vi "Inflation Apparatus.vi"() -> ()   [LabVIEW 2020]
uses:
  Inflation Test/Controls/Open Loop Controls.ctl
  Inflation Test/Controls/Ramp Controls.ctl
  Inflation Test/Controls/sinusoidal controls.ctl
  Inflation Test/Controls/Blood Pressure Controls.ctl
  Inflation Test/Controls/Hardware Options.ctl
  <vilib>/userdefined/High Color/IMAQdx.ctl
  Inflation Test/Controls/Common IA Test Control.ctl
  Controller Loop/Message and Data.ctl
  Inflation Test/Parameter Class/IA Test Parameters.lvclass
  Controllers/Controller.lvclass
  Hardware/Sensors/Cameras/Camera.lvclass
  Hardware/Sensors/Force Sensors/Force Sensor.lvclass
  Hardware/Actuators/Servos/Servo.lvclass
  Hardware/Actuators/Switches/Switch.lvclass
  Hardware/Sensors/Cameras/Camera.lvclass/Camera.ctl
  GUI/Main GUI Loop/Handler.ctl
  Hardware/Actuators/Switches/Switch.lvclass/Switch.ctl
  Hardware/Sensors/Cameras/USB Camera/USB Camera.lvclass
  C:/Users/jharw/Documents/1 Folder to Rule them All/UMD/Inflation-Apparatus/src/Hardware/Sensors/Cameras/Camera.lvclass
  Hardware/Sensors/Force Sensors/DAQmx Force Sensor/DAQmx Force Sensor.lvclass
  C:/Users/jharw/Documents/1 Folder to Rule them All/UMD/Inflation-Apparatus/src/Hardware/Sensors/Force Sensors/Force Sensor.lvclass
  Hardware/Actuators/Servos/DAQmx Servo/DAQmx Servo.lvclass
  C:/Users/jharw/Documents/1 Folder to Rule them All/UMD/Inflation-Apparatus/src/Hardware/Actuators/Servos/Servo.lvclass
  Hardware/Actuators/Switches/DAQmx Switch/DAQmx Switch.lvclass
  C:/Users/jharw/Documents/1 Folder to Rule them All/UMD/Inflation-Apparatus/src/Hardware/Actuators/Switches/Switch.lvclass
panel:
  in  "test equipment switch":bool
  in  "camera calibration switch":bool
  in  "force calibration switch":bool
  in  "inflation test switch":bool=TRUE
  in  "common test control":T1={"time delay (sec)"=2.0, "test time (sec)"=10.0, "diameter abort (mm)"=70.0, "sample rate (n/sec)"=30.0}
  in  "setpoint functions":T2(tab)
  in  "ramp controls":T3={"systole"=0.8, "diastole"=0.2}
  in  "sinusoidal controls":T4
  in  "blood-pressure controls":T5={"systole"=0.8, "systole 2"=0.2, "systole 3"=1.0, "systole 4"=0.6}
  in  "open-loop controls":T6={"high pw"=5.0, "low pw"=5.8}
  in  "base file name":string="test"
  in  "hardware controls":T7={"fs chan"="", "servo chan"="", "led chan"="", "camera port"="", "cam freq"=30.0, "fs freq"=30.0, "color pane"=0, "servo freq"=0.0} {"color pane" items=["Blue", "Red", "Green", "Saturation", "Value", "Intensity", "Luminance", "Hue", ""]}
  in  "folder path":path=path "C:/"
  in  "refresh hw?":bool caption="REFRESH?"
  in  "dynamic controls":T9(tab)
  out "camera framerate":dbl(knob)=9.99033583290062 caption="CAMERA FRAMERATE" scale=0.0..60.0
  in  "clear charts":bool
  in  "save to file":bool
  out "end time":timestamp caption="END TIME" format="%<%x %.3X>T"
  out "start time":timestamp caption="START TIME" format="%<%x %.3X>T"
  in  "abort test":bool
  in  "start test":bool
  in  "log force cal":bool
  in  "save force cal":bool
  in  "clear force cal":bool
  in  "update cal image":bool
  in  "launch va":bool
  in  "select cam cal":bool
  out "led status":bool
  in  "led switch":bool
  in  "dynamic indicators":T10(tab)
  out "force calibration results":dbl[][](array[numeric])
  out "force calibration array":dbl[][](array[numeric])
  in  "test cal":bool
  out "current diameter":dbl(graph)
  out "status":string
  out "version":string
  # "SETPOINT:"
  # "TIME DELAY (SEC):"
  # "TEST TIME (SEC):"
  # "TEST FREQUENCY (HZ):"
  # "DIAMETER ABORT (MM):"
  # "SETPOINT:"
  # "SYSTOLE (V):"
  # "DIASTOLE (V):"
  # "SETPOINT:"
  # "SYSTOLE (V):"
  # "DIASTOLE (V):"
  # "FREQUENCY (HZ):"
  # "SETPOINT:"
  # "SYSTOLE (V):"
  # "DIASTOLE (V):"
  # "DICROTIC NOTCH (V):"
  # "FREQUENCY (HZ):"
  # "SETPOINT:"
  # "HIGH PW (%):"
  # "LOW PW (%):"
  # "FOLDER PATH"
  # "BASE FILENAME"
  # "HARDWARE"
  # "FORCE SENSOR CHANNEL"
  # "SERVO CHANNEL"
  # "LED CHANNEL"
  # "CAMERA PORT"
  # "CAMERA FREQUENCY (HZ):"
  # "FS FREQUENCY (HZ):"
  # "SERVO FREQUENCY (HZ):"
  # "COLOR PANE:"
  # "TEST LED"
  # "TEST NUMBER"
  # "SLOPE (g/V)"
  # "INTERCEPT (g)"
  # "1"
  # "2"
  # "3"
  # "4"
  # "5"
  # "CALIBRATION RESULTS"
  # "TEST NUMBER"
  # "WEIGHT (GRAMS)"
  # "50"
  # "100"
  # "150"
  # "200"
  # "250"
  # "1"
  # "2"
  # "3"
  # "4"
  # "5"
  # "CALIBRATION VALUES (V)"
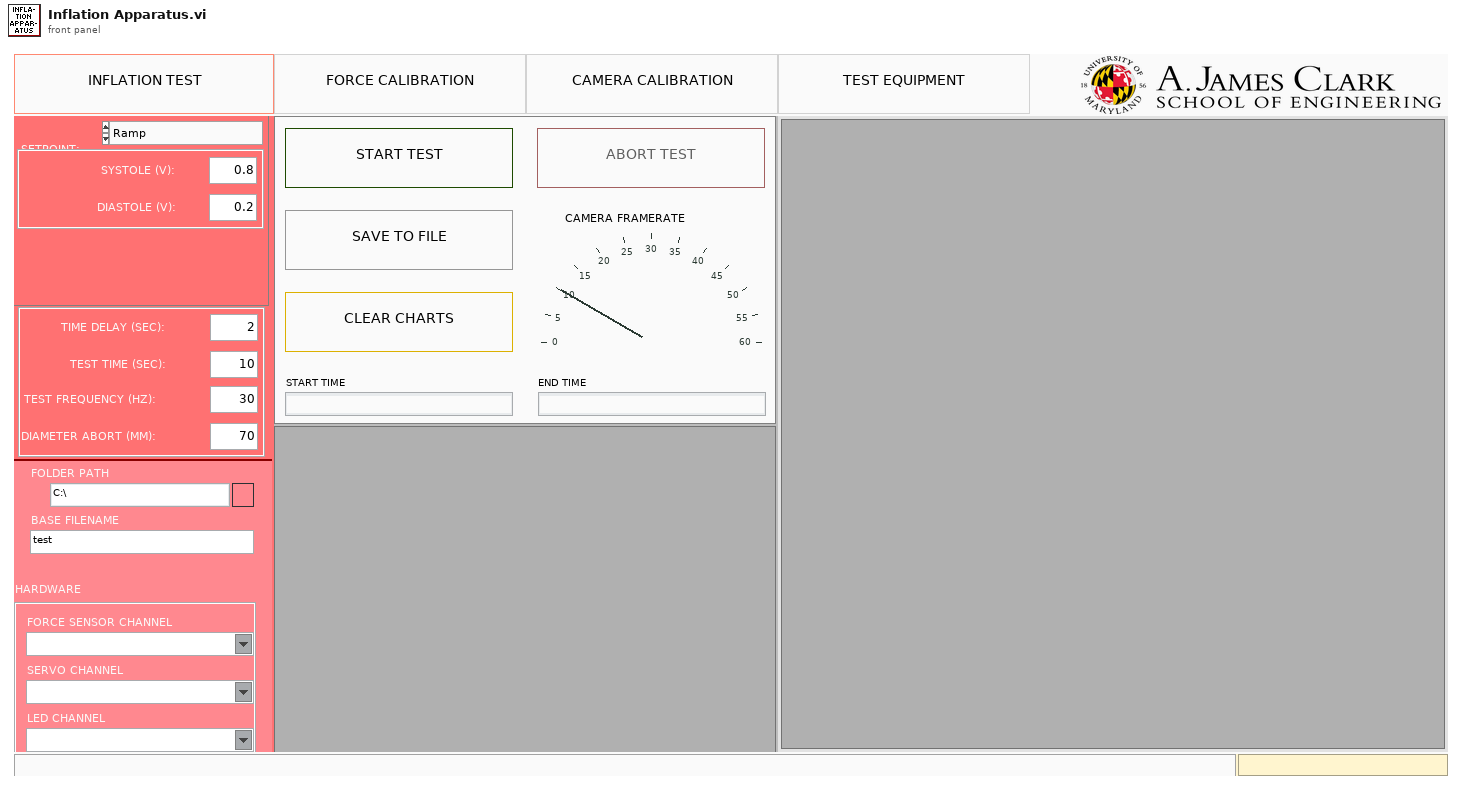
[diagram p1: front panel]
types:
  T1 = typedef "Common IA Test Control.ctl" = cluster{"time delay (sec)":dbl, "test time (sec)":dbl, "diameter abort (mm)":dbl, "sample rate (n/sec)":dbl}
  T2 = enum32{"Ramp", "Sinusoidal", "Blood-Pressure", "Open-Loop"}
  T3 = typedef "Ramp Controls.ctl" = cluster{"systole":dbl, "diastole":dbl}
  T4 = typedef "sinusoidal controls.ctl" = cluster{"systole":dbl, "systole 2":dbl, "systole 3":dbl}
  T5 = typedef "Blood Pressure Controls.ctl" = cluster{"systole":dbl, "systole 2":dbl, "systole 3":dbl, "systole 4":dbl}
  T6 = typedef "Open Loop Controls.ctl" = cluster{"high pw":dbl, "low pw":dbl}
  T7 = typedef "Hardware Options.ctl" = cluster{"fs chan":tag, "servo chan":tag, "led chan":tag, "camera port":T8, "cam freq":dbl, "fs freq":dbl, "color pane":i32, "servo freq":dbl}
  T8 = typedef "IMAQdx.ctl" = refnum<k21>
  T9 = enum32{"inflation test", "force calibration", "camera calibration", "test equipment"}
  T10 = enum32{"inflation test", "force calibration", "camera calibration"}
  T11 = typedef "Message and Data.ctl" = cluster{"msg":string, "ia test param":refnum<class "IA Test Parameters.lvclass">, "controller type":refnum<class "Controller.lvclass">, "folder path":path, "file name":string, "file comments":string, "cam":refnum<class "Camera.lvclass">, "fs":refnum<class "Force Sensor.lvclass">, "servo":refnum<class "Servo.lvclass">, "switch":refnum<class "Switch.lvclass">}
  T12 = typedef "Messaging Cluster.ctl" = cluster{"cam queue":refnum<queue>, "fs queue":refnum<queue>, "servo queue":refnum<queue>, "switch queue":refnum<queue>, "switch notifier":refnum<notifier>, "servo notifier":refnum<notifier>, "fs notifier":refnum<notifier>, "cam notifier":refnum<notifier>, "rgst evnt":refnum<event-registration>, "user event":refnum<user-event>, "ctlr queue":refnum<queue>, "main gui queue":refnum<queue>, "gui notifier":refnum<notifier>, "ia test notifier":refnum<notifier>}
  T13 = typedef "Tab Reference.ctl" = cluster{"dynamic controls":refnum<vi>, "dynamic indicators":refnum<vi>}
  T14 = typedef "GUI References.ctl" = cluster{"control tab":enum32{"inflation test", "force calibration", "camera calibration", "test equipment"}, "indicator tab":enum32{"inflation test", "force calibration", "camera calibration", "test equipment"}, "subpanel vi":refnum<vi>, "banner switch":refnum<vi>}
  T15 = typedef "Handler.ctl" = cluster{"bool ref":refnum<vi>, "error":errorcluster, "msg":string, "status":string, "switch status":bool, "force cal":dbl[][], "force cal results":dbl[][]}
  T16 = enum16{"Always On", "Always Off", "Off While Running"}
  T17 = enum8{"Enabled", "Disabled", "Disabled and Grayed Out"}
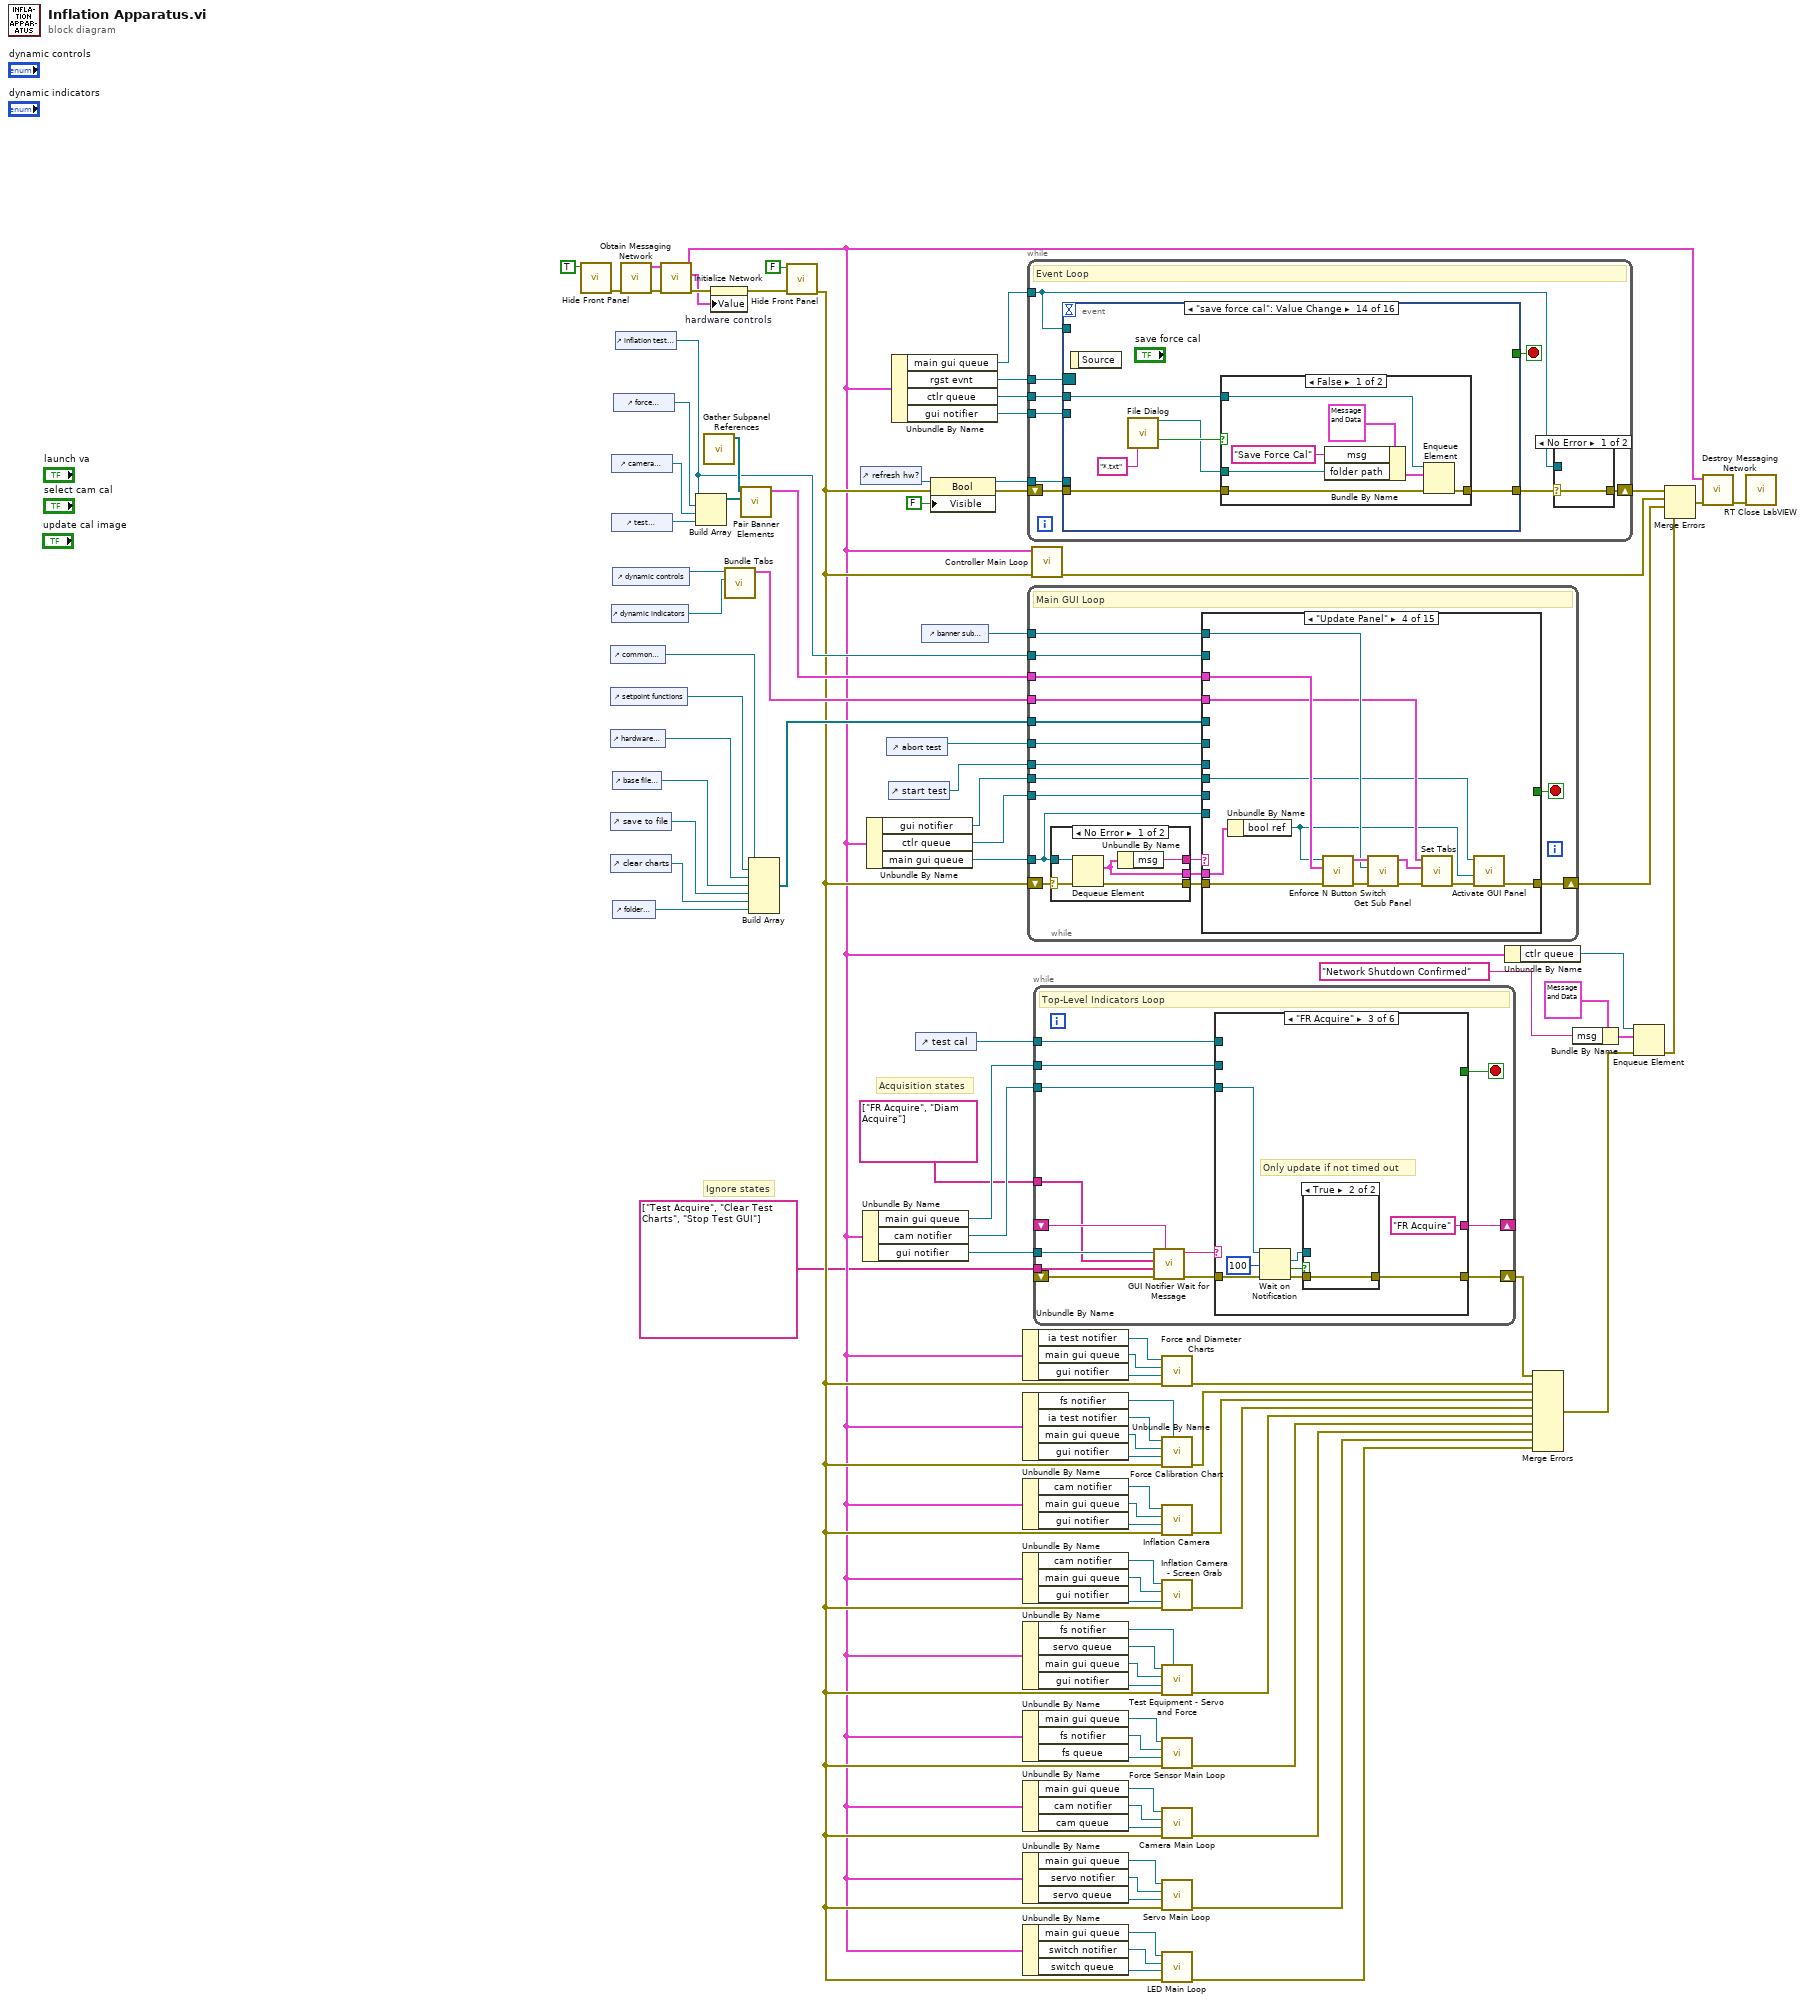
[diagram p0: block diagram]
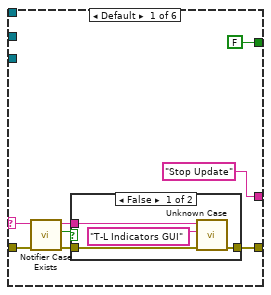
[diagram p2: hidden frame]
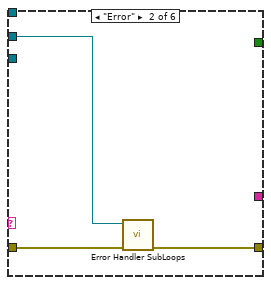
[diagram p4: hidden frame]
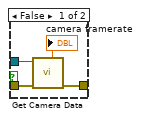
[diagram p5: hidden frame]
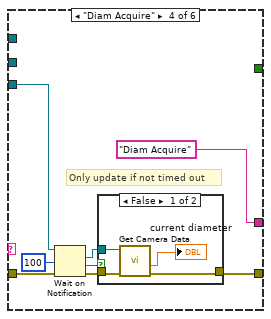
[diagram p6: hidden frame]
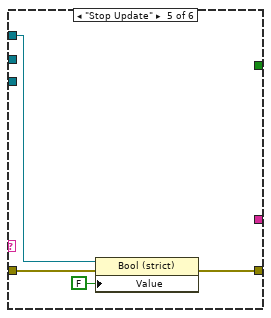
[diagram p8: hidden frame]
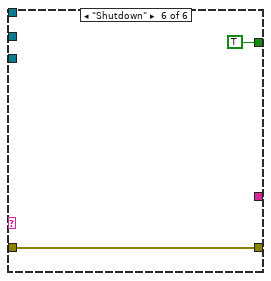
[diagram p9: hidden frame]
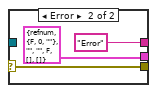
[diagram p10: hidden frame]
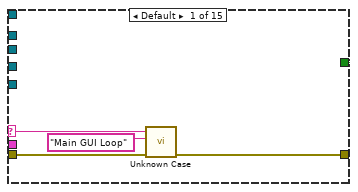
[diagram p11: hidden frame]
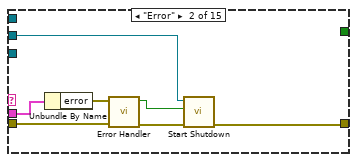
[diagram p12: hidden frame]
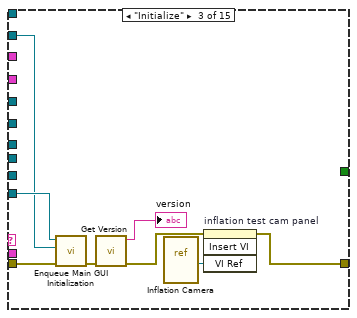
[diagram p13: hidden frame]
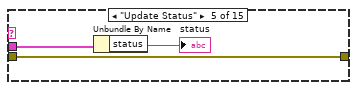
[diagram p14: hidden frame]
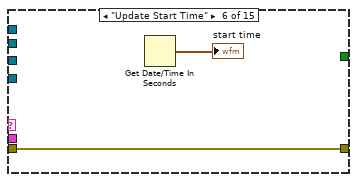
[diagram p15: hidden frame]
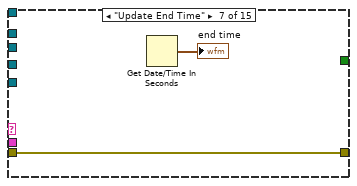
[diagram p16: hidden frame]
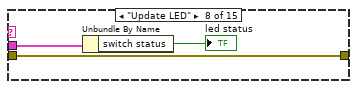
[diagram p17: hidden frame]
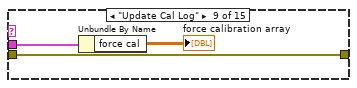
[diagram p18: hidden frame]
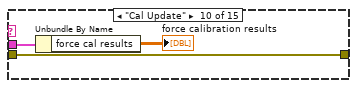
[diagram p19: hidden frame]
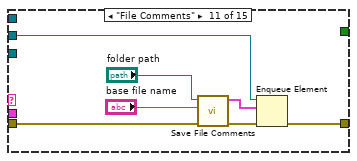
[diagram p20: hidden frame]
diagram:
  # "Ignore states"
  # "Acquisition states"
  n1 = call "Hide Front Panel.vi"("Hide IA Front Panel?"=TRUE ("Front Panel Window:Run VI Transparently")) -> ("error out"=w12:errorcluster)  [unwired: 10 in]
  n2 = control-ref of="common test control"() -> (w28:refnum<vi>)
  n3 = control-ref of="setpoint functions"() -> (w27:refnum<vi>)
  n4 = control-ref of="hardware controls"() -> (w29:refnum<vi>)
  n5 = control-ref of="save to file"() -> (w30:refnum<vi>)
  n6 = control-ref of="clear charts"() -> (w31:refnum<vi>)
  n7 = control-ref of="camera calibration switch"() -> (w98:refnum<vi>)
  n8 = control-ref of="test equipment switch"() -> (w96:refnum<vi>)
  n9 = control-ref of="dynamic indicators"() -> (w89:refnum<vi>)
  n10 = control-ref of="dynamic controls"() -> (w90:refnum<vi>)
  n11 = control-ref of="base file name"() -> (w19:refnum<vi>)
  n12 = control-ref of="folder path"() -> (w32:refnum<vi>)
  n13 = control-ref of="force calibration switch"() -> (w97:refnum<vi>)
  n14 = control-ref of="inflation test switch"() -> (w33:refnum<vi>)
  n15 = call "Obtain Messaging Network.vi"("error in (no error)"=w12) -> ("error out"=w13:errorcluster, "msg cluster"=w35:T12)  [unwired: 9 in]
  n16 = call "Initialize Network.vi"("error in (no error)"=w13, "msg cluster in"=w35) -> ("error out"=w22:errorcluster, "hardware controls out"=w21:T7, "msg cluster out"=w9:T12)  [unwired: 7 in]
  n17 = Build Array(w33, w97, w98, w96) -> (w91:refnum<vi>[])
  n18 = call "Gather Subpanel References.vi"() -> ("subpanel array"=w92:refnum<vi>[])  [unwired: 11 in]
  n19 = property on="hardware controls" class="Clust (strict)"(error in=w22, "Value"=w21) -> (error out=w16:errorcluster)  [unwired: 1 in, 1 out]
  n20 = call "Bundle Tabs.vi"("tab ref 2"=w89, "tab ref 1"=w90) -> ("tab references"=w76:T13)  [unwired: 9 in]
  n21 = call "Pair Banner Elements.vi"("boolean switch array in"=w91, "sub vi array in"=w92) -> ("banner gui refs"=w77:T14[])  [unwired: 9 in]
  n22 = Build Array(w28, w27, w29, w19, w30, w31, w32) -> (w26:refnum<vi>[])
  n23 = call "Hide Front Panel.vi"("error in (no error)"=w16, "Hide IA Front Panel?"=FALSE) -> ("error out"=w14:errorcluster)  [unwired: 9 in]
  n24 = control-ref of="refresh hw?"() -> (w95:refnum<vi>)
  n25 = Unbundle By Name(w9) -> ("main gui queue"=w8:refnum<queue>, "cam notifier"=w6:refnum<notifier>, "gui notifier"=w7:refnum<notifier>)
  n26 = Unbundle By Name(w9) -> ("gui notifier"=w10:refnum<notifier>, "ctlr queue"=w44:refnum<queue>, "main gui queue"=w88:refnum<queue>)
  n27 = control-ref of="abort test"() -> (w25:refnum<vi>)
  n28 = control-ref of="start test"() -> (w18:refnum<vi>)
  n29 = Unbundle By Name(w9) -> ("main gui queue"=w24:refnum<queue>, "rgst evnt"=w34:refnum<event-registration>, "ctlr queue"=w23:refnum<queue>, "gui notifier"=w20:refnum<notifier>)
  n30 = control-ref of="test cal"() -> (w4:refnum<vi>)
  n31 = control-ref of="banner sub panel"() -> (w78:refnum<vi>)
  n32 = property class="Bool"(reference=w95, error in=w14, "Visible"=FALSE) -> (reference out=w94:refnum<vi>, error out=w75:errorcluster)
  n33 = Unbundle By Name(w9) -> ("ia test notifier"=w72:refnum<notifier>, "main gui queue"=w70:refnum<queue>, "gui notifier"=w71:refnum<notifier>)
  n34 = Unbundle By Name(w9) -> ("fs notifier"=w1:refnum<notifier>, "ia test notifier"=w64:refnum<notifier>, "main gui queue"=w65:refnum<queue>, "gui notifier"=w66:refnum<notifier>)
  n35 = Unbundle By Name(w9) -> ("cam notifier"=w67:refnum<notifier>, "main gui queue"=w68:refnum<queue>, "gui notifier"=w69:refnum<notifier>)
  n36 = Unbundle By Name(w9) -> ("cam notifier"=w50:refnum<notifier>, "main gui queue"=w51:refnum<queue>, "gui notifier"=w52:refnum<notifier>)
  n37 = Unbundle By Name(w9) -> ("fs notifier"=w46:refnum<notifier>, "servo queue"=w47:refnum<queue>, "main gui queue"=w48:refnum<queue>, "gui notifier"=w49:refnum<notifier>)
  n38 = Unbundle By Name(w9) -> ("main gui queue"=w82:refnum<queue>, "fs notifier"=w83:refnum<notifier>, "fs queue"=w84:refnum<queue>)
  n39 = Unbundle By Name(w9) -> ("main gui queue"=w87:refnum<queue>, "cam notifier"=w86:refnum<notifier>, "cam queue"=w85:refnum<queue>)
  n40 = Unbundle By Name(w9) -> ("main gui queue"=w43:refnum<queue>, "servo notifier"=w42:refnum<notifier>, "servo queue"=w41:refnum<queue>)
  n41 = Unbundle By Name(w9) -> ("main gui queue"=w36:refnum<queue>, "switch notifier"=w37:refnum<notifier>, "switch queue"=w38:refnum<queue>)
  n42 = while {
    shift-right: [w101] -> w81
    shift-left: w75 -> [w106]
    tunnel: w94 -> [w105]
    tunnel: w34 -> [w104]
    tunnel: w23 -> [w103]
    tunnel: w24 -> [w102]
    tunnel: w20 -> [w99]
    stop <- w107 stop-if-true
    # "Event Loop"
    n43 = event shown="[13] \"save force cal\": Value Change" {
      selector: w104 -> [_ _ _ _ _ _ _ _ _ _ _ _ _ _ _ _]
      dyn-events: _ -> [_ _ _ _ _ _ _ _ _ _ _ _ _ _ _ _]
      timeout: _ -> [_ _ _ _ _ _ _ _ _ _ _ _ _ _ _ _]
      tunnel: [FALSE ("abort test") _ TRUE ("abort test") _ _ _ _ _ _ _ _ _ _ _ _ _] -> w107
      tunnel: [w112 w120 w124 w130 w133 w138 w158 w183 w188 w198 w207 w209 w216 w230 w249 w255] -> w100
      tunnel: w106 -> [w113 w121 w124 w131 w134 w139 w144 w178 w193 w202 w208 w210 w217 w231 w246 w256]
      tunnel: w105 -> [_ _ _ _ _ w140 w142 _ _ _ _ _ _ _ _ _]
      tunnel: w102 -> [w114 _ _ w126 _ _ _ _ _ _ w206 _ _ _ _ _]
      tunnel: w103 -> [_ _ _ _ _ _ w157 w184 w192 w197 _ w211 w218 w228 w244 _]
      tunnel: w99 -> [_ _ _ _ _ _ _ _ _ w201 _ _ _ _ _ w254]
      event "test equipment switch", "force calibration switch", "camera calibration switch", "inflation test switch": Value Change {
        n44 = event-data() -> ("CtlRef"=w115:refnum<vi>)  [unwired: 1 in]
        n45 = Bundle By Name(cluster=T15 {"bool ref"=refnum, "error"={"status"=FALSE, "code"=0, "source"=""}, "msg"="", "status"="", "switch status"=FALSE, "force cal"=[], "force cal results"=[]} ("element"), "msg"="Update Panel", "bool ref"=w115) -> (w117:T15)
        n46 = Enqueue Element(queue=w114, element=w117, error in (no error)=w113) -> (error out=w112:errorcluster)  [unwired: 1 in, 2 out]
      }
      event Mouse Enter {
        n47 = event-data() -> ("PaneRef"=w123:refnum<vi>)  [unwired: 1 in]
        n48 = property class="Pane"(reference=w123, error in=w121, "VertScrollbarVisibility"=T16."Always On" ("Horizontal Scrollbar Visibility")) -> (error out=w120:errorcluster)  [unwired: 1 out]
      }
      event User Event {
        n49 = event-data() -> ()  [unwired: 1 in, 1 out]
      }
      event Panel Close? {
        n50 = event-data() -> ()  [unwired: 1 in, 1 out]
        n51 = Bundle By Name(cluster=T15 {"bool ref"=refnum, "error"={"status"=FALSE, "code"=0, "source"=""}, "msg"="", "status"="", "switch status"=FALSE, "force cal"=[], "force cal results"=[]} ("element"), "msg"="Confirm Shutdown") -> (w127:T15)
        n52 = Enqueue Element(queue=w126, element=w127, error in (no error)=w131) -> (error out=w130:errorcluster)  [unwired: 1 in, 2 out]
        n53 = event-data("Discard?"=TRUE) -> ()  [unwired: 1 in, 1 out]
      }
      event Mouse Leave {
        n54 = event-data() -> ("PaneRef"=w136:refnum<vi>)  [unwired: 1 in]
        n55 = property class="Pane"(reference=w136, error in=w134, "VertScrollbarVisibility"=T16."Always Off" ("Horizontal Scrollbar Visibility")) -> (error out=w133:errorcluster)  [unwired: 1 out]
      }
      event Value Change {
        n56 = event-data() -> ()  [unwired: 1 in, 1 out]
        n57 = property class="Bool"(reference=w140, error in=w139, "Visible"=TRUE) -> (error out=w138:errorcluster)  [unwired: 1 out]
      }
      event "refresh hw?": Value Change {
        n58 = event-data() -> ()  [unwired: 1 in, 1 out]
        n59 = property class="Bool"(reference=w142, error in=w144, "Visible"=FALSE) -> (error out=w143:errorcluster)  [unwired: 1 out]
        n60 = call "HW Cluster to Classes.vi"("error in (no error)"=w143, "real hardware controls"="hardware controls") -> ("error out"=w154:errorcluster, "DAQmx Switch out"=w153:refnum<class "DAQmx Switch.lvclass">, "DAQmx Servo out"=w152:refnum<class "DAQmx Servo.lvclass">, "DAQmx Force Sensor out"=w151:refnum<class "DAQmx Force Sensor.lvclass">, "USB Camera out"=w150:refnum<class "USB Camera.lvclass">)  [unwired: 5 in]
        n61 = call "Check for DAQmx Errors.vi"("USB Camera in"=w150, "error in (no error)"=w154, "DAQmx Switch in"=w153, "DAQmx Servo in"=w152, "DAQmx Force Sensor in"=w151) -> ("error out"=w155:errorcluster, "DAQmx Switch out"=w149:refnum<class "DAQmx Switch.lvclass">, "DAQmx Servo out"=w148:refnum<class "DAQmx Servo.lvclass">, "DAQmx Force Sensor out"=w147:refnum<class "DAQmx Force Sensor.lvclass">, "USB Camera out"=w146:refnum<class "USB Camera.lvclass">)  [unwired: 2 in]
        n62 = call "Display Hardware Error.vi"("error in (no error)"=w155) -> ("error out"=w145:errorcluster, "Continue?"=w141:bool)  [unwired: 9 in]
        n63 = case shown="True" w141 {
          tunnel: [w160 w170] -> w158
          tunnel: w157 -> [_ w169]
          tunnel: w149 -> [_ w165]
          tunnel: w148 -> [_ w164]
          tunnel: w147 -> [_ w163]
          tunnel: w146 -> [_ w162]
          tunnel: w145 -> [w160 w161]
          frame False {
          }
          frame True {
            n64 = Bundle By Name(cluster=T11 {"msg"="", "ia test param"=refnum, "controller type"=refnum, "folder path"=path "", "file name"="", "file comments"="", "cam"=refnum, "fs"=refnum, "servo"=refnum, "switch"=refnum} ("element"), "msg"="Refresh HW", "cam"=w162, "fs"=w163, "servo"=w164, "switch"=w165) -> (w166:T11)
            n65 = Enqueue Element(queue=w169, element=w166, error in (no error)=w161) -> (error out=w170:errorcluster)  [unwired: 1 in, 2 out]
          }
        }
      }
      event "start test": Value Change {
        n66 = event-data() -> ()  [unwired: 1 in, 1 out]
        n67 = Format Into String("setpoint functions") -> (resulting string=w171:string)  [unwired: 3 in, 1 out]
        n68 = call "Set Setpoint Paramters.vi"("ramp controls"="ramp controls", "setpoint"=w171, "error in (no error)"=w178, "sinusoidal controls"="sinusoidal controls", "blood-pressure controls"="blood-pressure controls", "open-loop controls"="open-loop controls") -> ("error out"=w177:errorcluster, "IA test param out"=w179:refnum<class "IA Test Parameters.lvclass">)  [unwired: 4 in]
        n69 = call "Set Common Parameters.vi"("error in (no error)"=w177, "common test control"="common test control", "IA Test Parameters in"=w179) -> ("error out"=w182:errorcluster, "IA Test Parameters out"=w181:refnum<class "IA Test Parameters.lvclass">)  [unwired: 7 in]
        n70 = Bundle By Name(cluster=T11 {"msg"="", "ia test param"=refnum, "controller type"=refnum, "folder path"=path "", "file name"="", "file comments"="", "cam"=refnum, "fs"=refnum, "servo"=refnum, "switch"=refnum} ("element"), "msg"="Init IA Test", "ia test param"=w181) -> (w185:T11)
        n71 = Enqueue Element(queue=w184, element=w185, error in (no error)=w182) -> (error out=w183:errorcluster)  [unwired: 1 in, 2 out]
      }
      event "abort test": Value Change {
        n72 = event-data() -> ()  [unwired: 1 in, 1 out]
        n73 = Bundle By Name(cluster=T11 {"msg"="", "ia test param"=refnum, "controller type"=refnum, "folder path"=path "", "file name"="", "file comments"="", "cam"=refnum, "fs"=refnum, "servo"=refnum, "switch"=refnum} ("element"), "msg"="abort") -> (w189:T11)
        n74 = Enqueue Element(queue=w192, element=w189, error in (no error)=w193) -> (error out=w188:errorcluster)  [unwired: 1 in, 2 out]
      }
      event "clear charts": Value Change {
        n75 = event-data() -> ()  [unwired: 1 in, 1 out]
        n76 = Send Notification(notification="Clear Test Charts", notifier=w201, error in (no error)=w202) -> (error out=w199:errorcluster)  [unwired: 1 out]
        n77 = Bundle By Name(cluster=T11 {"msg"="", "ia test param"=refnum, "controller type"=refnum, "folder path"=path "", "file name"="", "file comments"="", "cam"=refnum, "fs"=refnum, "servo"=refnum, "switch"=refnum} ("element"), "msg"="Clear Test Data") -> (w195:T11)
        n78 = Enqueue Element(queue=w197, element=w195, error in (no error)=w199) -> (error out=w198:errorcluster)  [unwired: 1 in, 2 out]
      }
      event "save to file": Value Change {
        n79 = event-data() -> ()  [unwired: 1 in, 1 out]
        n80 = Bundle By Name(cluster=T15 {"bool ref"=refnum, "error"={"status"=FALSE, "code"=0, "source"=""}, "msg"="", "status"="", "switch status"=FALSE, "force cal"=[], "force cal results"=[]} ("element"), "msg"="File Comments") -> (w204:T15)
        n81 = Enqueue Element(queue=w206, element=w204, error in (no error)=w208) -> (error out=w207:errorcluster)  [unwired: 1 in, 2 out]
      }
      event "log force cal": Value Change {
        n82 = event-data() -> ()  [unwired: 1 in, 1 out]
        n83 = Bundle By Name(cluster=T11 {"msg"="", "ia test param"=refnum, "controller type"=refnum, "folder path"=path "", "file name"="", "file comments"="", "cam"=refnum, "fs"=refnum, "servo"=refnum, "switch"=refnum} ("element"), "msg"="Log Force Cal") -> (w213:T11)
        n84 = Enqueue Element(queue=w211, element=w213, error in (no error)=w210) -> (error out=w209:errorcluster)  [unwired: 1 in, 2 out]
      }
      event "clear force cal": Value Change {
        n85 = event-data() -> ()  [unwired: 1 in, 1 out]
        n86 = call "Confirm Clear Calibration.vi"() -> ("clear fs cal?"=w215:bool)  [unwired: 11 in]
        n87 = case shown="True" w215 {
          tunnel: w218 -> [_ w223]
          tunnel: w217 -> [w219 w221]
          tunnel: [w219 w220] -> w216
          frame False {
          }
          frame True {
            n88 = Bundle By Name(cluster=T11 {"msg"="", "ia test param"=refnum, "controller type"=refnum, "folder path"=path "", "file name"="", "file comments"="", "cam"=refnum, "fs"=refnum, "servo"=refnum, "switch"=refnum} ("element"), "msg"="Clear Force Cal") -> (w225:T11)
            n89 = Enqueue Element(queue=w223, element=w225, error in (no error)=w221) -> (error out=w220:errorcluster)  [unwired: 1 in, 2 out]
          }
        }
      }
      event "save force cal": Value Change {
        n90 = event-data() -> ()  [unwired: 1 in, 1 out]
        n91 = call "File Dialog"("pattern (all files)"="*.txt" ("pattern label")) -> ("selected path"=w227:path, "cancelled"=w229:bool)  [unwired: 11 in, 2 out]
        n92 = case shown="False" w229 {
          tunnel: w231 -> [w235 w239]
          tunnel: [w234 w239] -> w230
          tunnel: w228 -> [w233 _]
          tunnel: w227 -> [w232 _]
          frame False {
            n93 = Bundle By Name(cluster=T11 {"msg"="", "ia test param"=refnum, "controller type"=refnum, "folder path"=path "", "file name"="", "file comments"="", "cam"=refnum, "fs"=refnum, "servo"=refnum, "switch"=refnum} ("element"), "msg"="Save Force Cal", "folder path"=w232) -> (w238:T11)
            n94 = Enqueue Element(queue=w233, element=w238, error in (no error)=w235) -> (error out=w234:errorcluster)  [unwired: 1 in, 2 out]
          }
          frame True {
            # "Do nothing if cancelled"
          }
        }
      }
      event "led switch": Value Change {
        n95 = event-data() -> ()  [unwired: 1 in, 1 out]
        n96 = call "Set Switch State.vi"("error in (no error)"=w246, "switch state"="led switch", "Switch in"=refnum<class "Switch.lvclass"> refnum) -> ("error out"=w245:errorcluster, "Switch out"=w241:refnum<class "Switch.lvclass">)  [unwired: 7 in]
        n97 = Bundle By Name(cluster=T11 {"msg"="", "ia test param"=refnum, "controller type"=refnum, "folder path"=path "", "file name"="", "file comments"="", "cam"=refnum, "fs"=refnum, "servo"=refnum, "switch"=refnum} ("element"), "msg"="Actuate Switch", "switch"=w241) -> (w242:T11)
        n98 = Enqueue Element(queue=w244, element=w242, error in (no error)=w245) -> (error out=w249:errorcluster)  [unwired: 1 in, 2 out]
      }
      event "test cal": Value Change {
        n99 = event-data() -> ()  [unwired: 1 in, 1 out]
        n100 = Select(t="Diam Acquire" ("notification"), s="test cal", f="Stop Update") -> (s? t:f=w252:string)
        n101 = Send Notification(notification=w252, notifier=w254, error in (no error)=w256) -> (error out=w255:errorcluster)  [unwired: 1 out]
      }
    }
    n102 = case shown="No Error" w100 {
      selector: w100 -> [w108 w109]
      tunnel: w102 -> [_ w111]
      tunnel: [w108 w110] -> w101
      frame No Error {
      }
      frame Error {
        n103 = call "Error Handler SubLoops.vi"("error in"=w109, "main gui queue"=w111) -> ("error out"=w110:errorcluster)  [unwired: 9 in]
      }
    }
  }
  n104 = while {
    shift-right: [w268] -> w73
    shift-left: w14 -> [w272]
    tunnel: w88 -> [w262]
    tunnel: w78 -> [w266]
    tunnel: w77 -> [w265]
    tunnel: w33 -> [w264]
    tunnel: w76 -> [w263]
    tunnel: w44 -> [w261]
    tunnel: w26 -> [w260]
    tunnel: w25 -> [w259]
    tunnel: w18 -> [w258]
    tunnel: w10 -> [w257]
    stop <- w267 stop-if-true
    # "Main GUI Loop"
    n105 = case shown="No Error" w272 {
      selector: w272 -> [w276 w280]
      tunnel: [w277 w280] -> w269
      tunnel: w262 -> [w275 _]
      tunnel: [w274 "Error" ("msg")] -> w270
      tunnel: [w273 T15 {"bool ref"=refnum, "error"={"status"=FALSE, "code"=0, "source"=""}, "msg"="", "status"="", "switch status"=FALSE, "force cal"=[], "force cal results"=[]} ("main gui")] -> w271
      frame No Error {
        n106 = Dequeue Element(queue=w275, error in (no error)=w276) -> (element=w273:T15, error out=w277:errorcluster)  [unwired: 1 in, 2 out]
        n107 = Unbundle By Name(w273) -> ("msg"=w274:string)
      }
      frame Error {
      }
    }
    n108 = case shown="\"Update Panel\"" w270 {
      selector: w270 -> [w283 _ _ _ _ _ _ _ _ _ _ _ _ _ _]
      tunnel: w271 -> [_ w289 _ w309 w316 _ _ w323 w326 w329 _ _ _ _ _]
      tunnel: w269 -> [w285 w292 w298 w313 w314 w318 w319 w321 w324 w327 w334 w341 w357 w372 w374]
      tunnel: [w284 w290 w293 w303 w314 w318 w319 w321 w324 w327 w336 w349 w363 w371 w374] -> w268
      tunnel: [FALSE _ _ _ _ _ _ _ _ _ _ _ _ _ TRUE] -> w267
      tunnel: w266 -> [_ _ _ w307 _ _ _ _ _ _ _ _ _ _ _]
      tunnel: w265 -> [_ _ _ w308 _ _ _ _ _ _ _ w345 w361 _ _]
      tunnel: w264 -> [_ _ w295 _ _ _ _ _ _ _ _ _ _ _ _]
      tunnel: w263 -> [_ _ _ w305 _ _ _ _ _ _ _ _ _ _ _]
      tunnel: w262 -> [_ _ w296 _ _ _ _ _ _ _ _ _ _ _ _]
      tunnel: w261 -> [_ w286 _ _ _ _ _ _ _ _ w335 _ _ w373 _]
      tunnel: w260 -> [_ _ _ _ _ _ _ _ _ _ _ w343 w360 _ _]
      tunnel: w259 -> [_ _ _ _ _ _ _ _ _ _ _ w347 w367 _ _]
      tunnel: w258 -> [_ _ _ _ _ _ _ _ _ _ _ w339 w358 _ _]
      tunnel: w257 -> [_ _ _ w301 _ _ _ _ _ _ _ _ _ _ _]
      frame Default {
        n109 = call "Unknown Case.vi"("error in (no error)"=w285, "source"="Main GUI Loop", "case"=w283) -> ("error out"=w284:errorcluster)  [unwired: 8 in]
      }
      frame "Error" {
        n110 = Unbundle By Name(w289) -> ("error"=w288:errorcluster)
        n111 = call "Error Handler.vi"("error in (no error)"=w292, "other error"=w288) -> ("error out"=w291:errorcluster, "stop program?"=w287:bool)  [unwired: 8 in]
        n112 = call "Start Shutdown.vi"("error in (no error)"=w291, "stop application?"=w287, "controller queue"=w286) -> ("error out"=w290:errorcluster)  [unwired: 8 in]
      }
      frame "Initialize" {
        n113 = call "Enqueue Main GUI Initialization.vi"("error in (no error)"=w298, "boolean reference"=w295, "main gui queue"=w296) -> ("error out"=w294:errorcluster)  [unwired: 8 in]
        n114 = call "Get Version.vi"("error in (no error)"=w294) -> ("error out"=w300:errorcluster, "version"=→"version":string)  [unwired: 9 in]
        n115 = vi-ref "Inflation Camera.vi"() -> (w299:refnum<vi>)
        n116 = invoke on="inflation test cam panel" class="SubPnl" method="Insert VI"(error in=w300, "VI Ref"=w299) -> (error out=w293:errorcluster)  [unwired: 2 in, 3 out]
      }
      frame "Update Panel" {
        n117 = Unbundle By Name(w309) -> ("bool ref"=w302:refnum<vi>)
        n118 = call "Enforce N Button Switch.vi"("error in (no error)"=w313, "banner gui refs"=w308, "boolean reference in"=w302) -> ("error out"=w312:errorcluster, "selected gui pairing"=w310:T14)  [unwired: 7 in]
        n119 = call "Get Sub Panel.vi"("error in (no error)"=w312, "subpanel in"=w307, "selected gui pairing in"=w310) -> ("error out"=w311:errorcluster, "selected gui pairing out"=w306:T14)  [unwired: 7 in]
        n120 = call "Set Tabs.vi"("error in (no error)"=w311, "gui pairing"=w306, "tab references"=w305) -> ("error out"=w304:errorcluster)  [unwired: 8 in]
        n121 = call "Activate GUI Panel.vi"("error in (no error)"=w304, "banner ref"=w302, "gui notifier"=w301) -> ("error out"=w303:errorcluster)  [unwired: 8 in]
      }
      frame "Update Status" {
        n122 = Unbundle By Name(w316) -> ("status"=→"status":string)
      }
      frame "Update Start Time" {
        n123 = Get Date/Time In Seconds() -> (seconds since 1Jan1904=→"start time":timestamp)
      }
      frame "Update End Time" {
        n124 = Get Date/Time In Seconds() -> (seconds since 1Jan1904=→"end time":timestamp)
      }
      frame "Update LED" {
        n125 = Unbundle By Name(w323) -> ("switch status"=→"led status":bool)
      }
      frame "Update Cal Log" {
        n126 = Unbundle By Name(w326) -> ("force cal"=→"force calibration array":dbl[][])
      }
      frame "Cal Update" {
        n127 = Unbundle By Name(w329) -> ("force cal results"=→"force calibration results":dbl[][])
      }
      frame "File Comments" {
        n128 = call "Save File Comments.vi"("error in (no error)"=w334, "base file name"="base file name", "folder path"="folder path") -> ("error out"=w333:errorcluster, "controller data"=w332:T11)  [unwired: 7 in]
        n129 = Enqueue Element(queue=w335, element=w332, error in (no error)=w333) -> (error out=w336:errorcluster)  [unwired: 1 in, 2 out]
      }
      frame "Deactivate Test Panel" {
        n130 = for {
          tunnel: w345 -> [w353] mode=indexing
          tunnel: [w352] -> w344 mode=indexing
          n131 = Unbundle By Name(w353) -> ("banner switch"=w352:refnum<vi>)
        }
        n132 = Build Array(w347) -> (w346:refnum<vi>[])
        n133 = Build Array(w339) -> (w338:refnum<vi>[])
        n134 = call "Disable References.vi"("error in (no error)"=w341, "disable? enum"=T17."Disabled" ("Disabled"), "ref array"=w338) -> ("error out"=w340:errorcluster)  [unwired: 8 in]
        n135 = Build Array (concatenate)(w344, w343) -> (w342:refnum<vi>[])
        n136 = call "Disable References.vi"("error in (no error)"=w340, "disable? enum"=T17."Enabled", "ref array"=w346) -> ("error out"=w348:errorcluster)  [unwired: 8 in]
        n137 = call "Disable References.vi"("error in (no error)"=w348, "disable? enum"=T17."Disabled and Grayed Out" ("Disabled"), "ref array"=w342) -> ("error out"=w349:errorcluster)  [unwired: 8 in]
      }
      frame "Activate Test Panel" {
        n138 = for {
          tunnel: w361 -> [w370] mode=indexing
          tunnel: [w369] -> w362 mode=indexing
          n139 = Unbundle By Name(w370) -> ("banner switch"=w369:refnum<vi>)
        }
        n140 = Build Array(w367) -> (w366:refnum<vi>[])
        n141 = property class="Bool (strict)"(reference=w358, error in=w357, "Value"=FALSE ("start test"), "DisabledEnum"=T17."Enabled" ("Disabled")) -> (error out=w356:errorcluster)  [unwired: 1 out]
        n142 = call "Disable References.vi"("error in (no error)"=w356, "disable? enum"=T17."Disabled and Grayed Out", "ref array"=w366) -> ("error out"=w364:errorcluster)  [unwired: 8 in]
        n143 = Build Array (concatenate)(w362, w360) -> (w359:refnum<vi>[])
        n144 = call "Disable References.vi"("error in (no error)"=w364, "disable? enum"=T17."Enabled" ("Disabled"), "ref array"=w359) -> ("error out"=w363:errorcluster)  [unwired: 8 in]
      }
      frame "Confirm Shutdown" {
        n145 = call "Confirm Shutdown.vi"("error in (no error)"=w372, "controller queue"=w373) -> ("error out"=w371:errorcluster)  [unwired: 9 in]
      }
      frame "Shutdown" {
      }
    }
  }
  n146 = call "Controller Main Loop.vi"("error in (no error)"=w14, "msg cluster"=w9) -> ("error out"=w74:errorcluster)  [unwired: 9 in]
  n147 = while {
    shift-right: [w387] -> w2
    shift-left: _ -> [w384]
    tunnel: w8 -> [w386]
    shift-right: [w385] -> _
    shift-left: _ -> [w382]
    tunnel: w7 -> [w381]
    tunnel: w6 -> [w380]
    tunnel: string[] ["FR Acquire", "Diam Acquire"] ("t") -> [w379]
    tunnel: string[] ["Test Acquire", "Clear Test Charts", "Stop Test GUI"] ("x") -> [w378]
    tunnel: w4 -> [w376]
    stop <- w388 stop-if-true
    # "Top-Level Indicators Loop"
    n148 = call "GUI Notifier Wait for Message.vi"("last state"=w382, "error in (no error)"=w384, "cases to ignore"=w378, "acquisition states"=w379, "gui notifier"=w381) -> ("error out"=w383:errorcluster, "gui msg"=w377:string)  [unwired: 5 in]
    n149 = case shown="\"FR Acquire\"" w377 {
      selector: w377 -> [w393 _ _ _ _ _]
      tunnel: [FALSE _ _ _ _ TRUE] -> w388
      tunnel: [w395 w404 w408 w421 w433 w435] -> w387
      tunnel: ["Stop Update" _ "FR Acquire" "Diam Acquire" _ _] -> w385
      tunnel: w386 -> [_ w403 _ _ _ _]
      tunnel: w383 -> [w389 w402 w409 w424 w434 w435]
      tunnel: w380 -> [_ _ w405 w423 _ _]
      tunnel: w376 -> [_ _ _ _ w432 _]
      frame Default {
        n150 = call "Notifier Case Exists.vi"("error in (no error)"=w389, "case in"=w393) -> ("error out"=w394:errorcluster, "defined case?"=w391:bool, "case out"=w392:string)  [unwired: 7 in]
        n151 = case shown="False" w391 {
          tunnel: [w400 w401] -> w395
          tunnel: w394 -> [w398 w401]
          tunnel: w392 -> [w397 _]
          frame False {
            n152 = call "Unknown Case.vi"("error in (no error)"=w398, "source"="T-L Indicators GUI", "case"=w397) -> ("error out"=w400:errorcluster)  [unwired: 8 in]
          }
          frame True {
          }
        }
      }
      frame "Error" {
        n153 = call "Error Handler SubLoops.vi"("error in"=w402, "main gui queue"=w403) -> ("error out"=w404:errorcluster)  [unwired: 9 in]
      }
      frame "FR Acquire" {
        # "Only update if not timed out"
        n154 = Wait on Notification(notifier=w405, timeout in ms (-1)=100, error in (no error)=w409) -> (notification=w411:refnum<class "Camera.lvclass">, timed out?=w406:bool, error out=w412:errorcluster)  [unwired: 1 in, 1 out]
        n155 = case shown="True" w406 {
          tunnel: w412 -> [w416 w417]
          tunnel: w411 -> [w415 _]
          tunnel: [w413 w417] -> w408
          frame False {
            n156 = call "Get Camera Data.vi"("error in (no error)"=w416, "Camera in"=w415) -> ("error out"=w413:errorcluster, "cam framerate (hz)"=→"camera framerate":dbl)  [unwired: 5 in, 3 out]
          }
          frame True {
          }
        }
      }
      frame "Diam Acquire" {
        # "Only update if not timed out"
        n157 = Wait on Notification(notifier=w423, timeout in ms (-1)=100, error in (no error)=w424) -> (notification=w419:refnum<class "Camera.lvclass">, timed out?=w420:bool, error out=w422:errorcluster)  [unwired: 1 in, 1 out]
        n158 = case shown="False" w420 {
          tunnel: w422 -> [w428 w430]
          tunnel: [w427 w430] -> w421
          tunnel: w419 -> [w426 _]
          frame False {
            n159 = call "Get Camera Data.vi"("error in (no error)"=w428, "Camera in"=w426) -> ("error out"=w427:errorcluster, "diameter (mm)"=→"current diameter":dbl)  [unwired: 5 in, 3 out]
          }
          frame True {
          }
        }
      }
      frame "Stop Update" {
        n160 = property class="Bool (strict)"(reference=w432, error in=w434, "Value"=FALSE) -> (error out=w433:errorcluster)  [unwired: 1 out]
      }
      frame "Shutdown" {
      }
    }
  }
  n161 = call "Force and Diameter Charts.vi"("error in (no error)"=w14, "gui notifier"=w71, "error queue"=w70, "ia test notifier"=w72) -> ("error out"=w63:errorcluster)  [unwired: 7 in]
  n162 = call "Force Calibration Chart.vi"("fs notifier"=w1, "error in (no error)"=w14, "gui notifier"=w66, "error queue"=w65, "ia test notifier"=w64) -> ("error out"=w62:errorcluster)  [unwired: 6 in]
  n163 = call "Inflation Camera.vi"("error in (no error)"=w14, "gui notifier"=w69, "error queue"=w68, "cam notifier"=w67) -> ("error out"=w61:errorcluster)  [unwired: 7 in]
  n164 = call "Inflation Camera - Screen Grab.vi"("error in (no error)"=w14, "gui notifier"=w52, "error queue"=w51, "cam notifier"=w50) -> ("error out"=w53:errorcluster)  [unwired: 7 in]
  n165 = call "Test Equipment - Servo and Force.vi"("fs notifier"=w46, "error in (no error)"=w14, "gui notifier"=w49, "error queue"=w48, "servo queue"=w47) -> ("error out"=w45:errorcluster)  [unwired: 6 in]
  n166 = call "Force Sensor Main Loop.vi"("error in (no error)"=w14, "fs queue"=w84, "fs notifier"=w83, "error queue"=w82) -> ("error out"=w60:errorcluster)  [unwired: 7 in]
  n167 = call "Camera Main Loop.vi"("error in (no error)"=w14, "cam queue"=w85, "cam notifier"=w86, "error queue"=w87) -> ("error out"=w59:errorcluster)  [unwired: 7 in]
  n168 = call "Servo Main Loop.vi"("error in (no error)"=w14, "servo queue"=w41, "servo notifier"=w42, "error queue"=w43) -> ("error out"=w40:errorcluster)  [unwired: 7 in]
  n169 = call "LED Main Loop.vi"("error in (no error)"=w14, "switch queue"=w38, "switch notifier"=w37, "main gui queue"=w36) -> ("error out"=w39:errorcluster)  [unwired: 7 in]
  n170 = Unbundle By Name(w9) -> ("ctlr queue"=w56:refnum<queue>)
  n171 = Merge Errors(w2, w63, w62, w61, w53, w45, w60, w59, w40, w39) -> (w58:errorcluster)
  n172 = Bundle By Name(cluster=T11 {"msg"="", "ia test param"=refnum, "controller type"=refnum, "folder path"=path "", "file name"="", "file comments"="", "cam"=refnum, "fs"=refnum, "servo"=refnum, "switch"=refnum} ("cntlr type"), "msg"="Network Shutdown Confirmed") -> (w55:T11)
  n173 = Enqueue Element(queue=w56, element=w55, error in (no error)=w58) -> (error out=w57:errorcluster)  [unwired: 1 in, 2 out]
  n174 = Merge Errors(w81, w74, w73, w57) -> (w80:errorcluster)
  n175 = call "Destroy Messaging Network.vi"("error in (no error)"=w80, "msg cluster"=w9) -> ("error out"=w79:errorcluster)  [unwired: 9 in]
  n176 = call "RT Close LabVIEW.vi"("error in (no error)"=w79) -> ()  [unwired: 10 in, 1 out]
